vi "Sequence for Constant Dragging with dragging.vi"() -> ()   [LabVIEW 2011]
doc: "The Sequence VI acquires a sequence of images and displays the images in an image control using high-level acquisition VIs. A sequence is appropriate for applications in which you want to process multiple images."
uses:
  <vilib>/userDefined/High Color/IMAQdx.ctl
  <vilib>/vision/driver/IMAQdx.llb/IMAQdx Acquisition Mode.ctl
  <vilib>/Platform/TimedLoop/XDataNode/timing_clust.ctl
  <vilib>/Platform/TimedLoop/XDataNode/nitl_modes.ctl
  <vilib>/Platform/TimedLoop/XDataNode/wakeup.ctl
  <vilib>/vision/driver/IMAQdx.llb/IMAQdx Buffer Number Mode.ctl
  <vilib>/Platform/TimedLoop/XDataNode/XDataNode.xnode
  <vilib>/vision/driver/NI_Vision_Acquisition_Software.lvlib
  Program Files/National Instruments/LabVIEW 2011/resource/objmgr/imaqdx.rc
  <vilib>/Platform/TimedLoop/XDataNode/XDNodeRunTimeDep.lvlib
  Program Files/Mad City Labs/NanoDrive/Madlib.dll
panel:
  in  "Drag Speed (um/s)":dbl min=0.0 step=0.01 format="%_3g"
  in  "Handle 2":i32
  in  "Exposure (us)":dbl(slide)=1407.017543859649 min=100.0 max=15000.0 step=100.0 scale=100.0..15000.0
  out "Acquisition  progress":i32(slide) scale=0.0..10999.0
  in  "BitsPerPixel":u32(ring) items=["Use Hardware Value"=0, "10-bit"=10, "12-bit"=12, "14-bit"=14, "16-bit"=16]
  in  "Height":u32=1080
  in  "Width":u32=1920
  in  "Number of Frames":u32=250
  in  "Frame Rate":dbl=55.0
  in  "Path":path
  in  "Camera Name":T1
  out "Image Array":T2[](array[plugin-control])
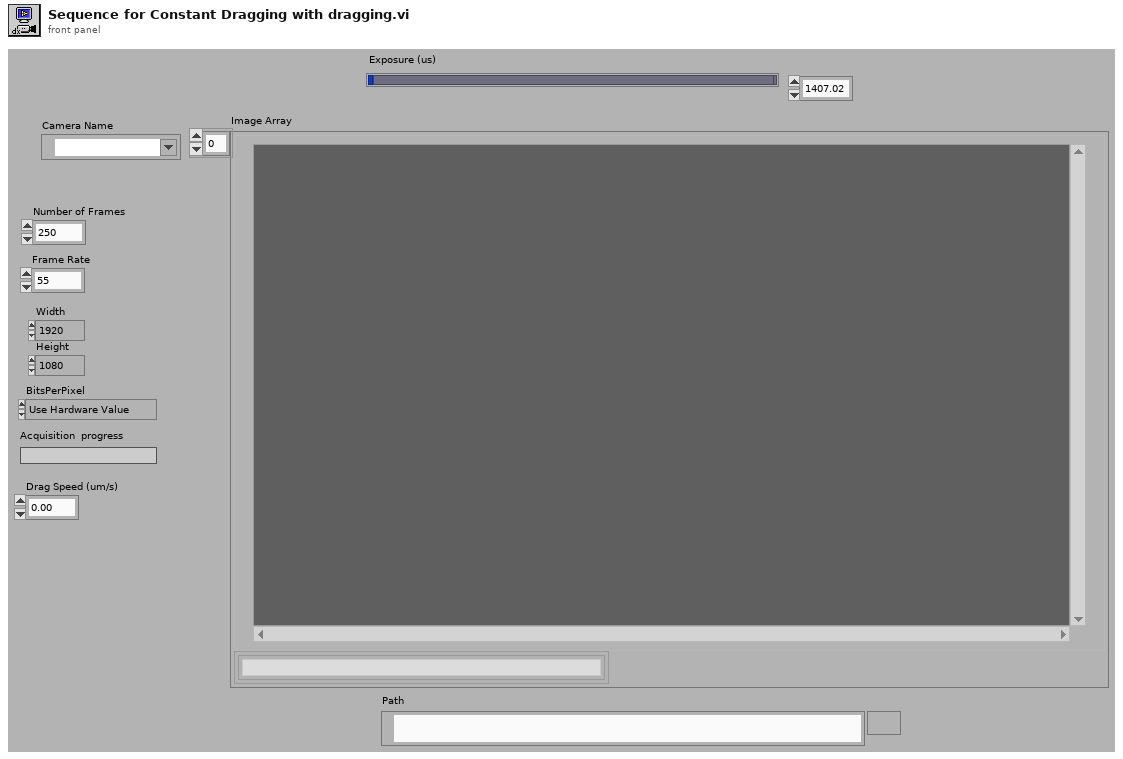
[diagram p1: front panel]
types:
  T1 = typedef "IMAQdx.ctl" = refnum<k21>
  T2 = typedef "IMAQ Image.ctl" = refnum<image>
  T3 = typedef "NI_Vision_Acquisition_Software.lvlib/IMAQdx Acquisition Mode.ctl" = enum32{"One Shot", "Continuous"}
  T4 = typedef "XDNodeRunTimeDep.lvlib/timing_clust.ctl" = cluster{"Expected End [f-1]":u64, "Actual End [f-1]":u64, "Finished Late? [f-1]":bool, "Expected End [i-1]":u64, "Actual End [i-1]":u64, "Finished Late? [i-1]":bool, "Expected Start [i]":u64, "Actual Start [i]":u64, "Expected Start [f]":u64, "Actual Start [f]":u64, "Source Name":string, "Structure Name":string, "Period":i64, "Deadline":i64, "Offset":i64, "Start":i64, "Priority":i32, "Timeout":i32, "Mode":T5, "Wakeup Reason":T6, "Error":errorcluster, "Source Type":string, "Secondary Source Type":string, "Global End Time":u64, "Global Start Time":u64, "Frame Duration":u64, "Iteration Duration":u64, "Assigned CPU":i32, "I/O Scan Engine Mode":u32}
  T5 = typedef "XDNodeRunTimeDep.lvlib/nitl_modes.ctl" = enum32{"No Change", "Process missed periods, maintain original phase", "Discard missed periods, maintain original phase", "Process missed periods, ignore original phase", "Discard missed periods, ignore original phase"}
  T6 = typedef "XDNodeRunTimeDep.lvlib/wakeup.ctl" = enum32{"Normal", "Aborted", "Asynchronous wakeup", "Timing source error", "Timed loop error", "Timeout"}
  T7 = typedef "NI_Vision_Acquisition_Software.lvlib/IMAQdx Buffer Number Mode.ctl" = enum32{"Next", "Last", "Buffer Number"}
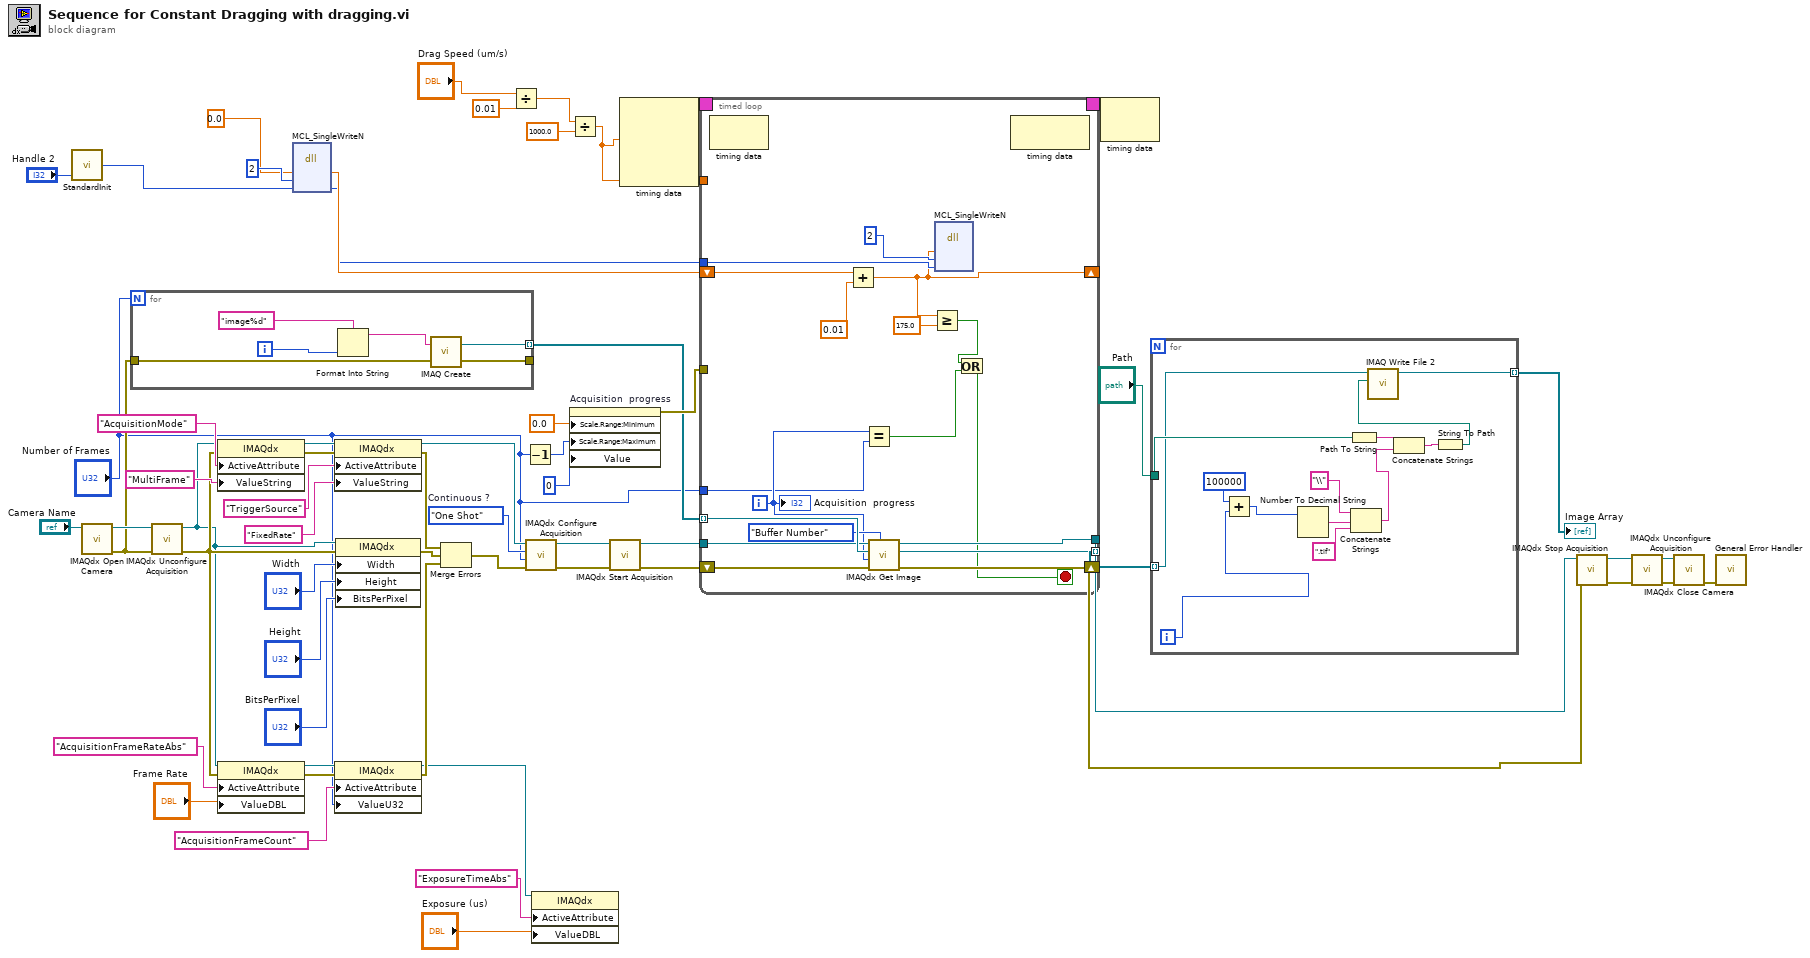
[diagram p0: block diagram]
diagram:
  w38 = IMAQdx_Acquisition_Mode."One Shot"  # Continuous ?
  n1 = call "StandardInit.vi"("Incoming Handle"="Handle 2") -> ("Outgoing Handle"=w11:i32)
  n2 = call <vilib>:"IMAQdx Open Camera.vi"("Session In"="Camera Name") -> ("error out"=w48:errorcluster, "Session Out"=w49:T1)  [unwired: 2 in, 7 out]
  n3 = for {
    N: "Number of Frames" -> [_]
    tunnel: w48 -> [w67]
    tunnel: [w66] -> w26 mode=indexing
    tunnel: [w65] -> _
    i -> [w64]
    n4 = Format Into String(format string="image%d" ("Image Name"), w64) -> (resulting string=w63:string)  [unwired: 2 in, 1 out]
    n5 = call "IMAQ Create"("Image Name"=w63, "error in (no error)"=w67) -> ("New Image"=w66:T2, "error out"=w65:errorcluster)  [unwired: 2 in, 1 out]
  }
  n6 = call <vilib>:"IMAQdx Unconfigure Acquisition.vi"("error in"=w48, "Session In"=w49) -> ("error out"=w43:errorcluster, "Session Out"=w40:T1)  [unwired: 8 out]
  n7 = property class="IMAQdx"(reference=w40, error in=w43, "ActiveAttribute"="AcquisitionMode", "ValueString"="MultiFrame") -> (reference out=w44:T1, error out=w54:errorcluster)
  n8 = property class="IMAQdx"(reference=w40, error in=w43, "ActiveAttribute"="AcquisitionFrameRateAbs", "ValueDBL"="Frame Rate") -> (reference out=w58:T1, error out=w57:errorcluster)
  n9 = dll-call lib="C:/Program Files/Mad City Labs/NanoDrive/Madlib.dll" fn="MCL_SingleWriteN"("position"=0.0, "axis"=u32 2, "handle"=w11) -> ("position"=w5:dbl, "handle"=w4:i32)  [unwired: 4 in, 3 out]
  n10 = property class="IMAQdx"(reference=w44, error in=w54, "ActiveAttribute"="TriggerSource", "ValueString"="FixedRate") -> (reference out=w25:T1, error out=w50:errorcluster)
  n11 = property class="IMAQdx"(reference=w58, error in=w57, "ActiveAttribute"="AcquisitionFrameCount", "ValueU32"="Number of Frames") -> (reference out=w15:T1, error out=w51:errorcluster)
  n12 = property class="IMAQdx"(reference=w40, error in=w43, "Width"="Width", "Height"="Height", "BitsPerPixel"="BitsPerPixel") -> (error out=w42:errorcluster)  [unwired: 1 out]
  n13 = Merge Errors(w50, w42, w51) -> (w22:errorcluster)
  n14 = Divide(x="Drag Speed (um/s)", y=0.01) -> (x/y=w7:dbl)
  n15 = Decrement(x="Number of Frames") -> (x-1=w35:u32)
  n16 = call <vilib>:"IMAQdx Configure Acquisition.vi"("error in"=w22, "Number of Buffers"="Number of Frames", "Continuous?"=w38, "Session In"=w25) -> ("error out"=w21:errorcluster, "Session Out"=w24:T1)  [unwired: 6 out]
  n17 = property class="IMAQdx"(reference=w15, "ActiveAttribute"="ExposureTimeAbs", "ValueDBL"="Exposure (us)") -> ()  [unwired: 1 in, 2 out]
  n18 = Divide(x=w7, y=1000.0) -> (x/y=w1:dbl)
  n19 = property on="Acquisition  progress" class="Slide (strict)"("Scale.Range:Minimum"=0.0 ("Write Attribute"), "Scale.Range:Maximum"=w35, "Value"=u32 0 ("Acquisition  progress")) -> (error out=w27:errorcluster)  [unwired: 2 in, 1 out]
  n20 = call <vilib>:"IMAQdx Start Acquisition.vi"("error in"=w21, "Session In"=w24) -> ("error out"=w37:errorcluster, "Session Out"=w23:T1)  [unwired: 8 out]
  n21 = node-c288(w1) -> (w3:T4)  [unwired: 3 in]
  n22 = timed-loop {
    tunnel: w26 -> [w85] mode=indexing
    shift-right: [w83] -> w34
    shift-left: w37 -> [w84]
    tunnel: [w82] -> w33
    tunnel: w23 -> [w81]
    tunnel: [w79] -> w19 mode=indexing
    tunnel: w27 -> [_]
    tunnel: "Number of Frames" -> [w77]
    tunnel: w1 -> [_]
    tunnel: w4 -> [w76]
    timing: w3 -> [_]
    timing-out: [_] -> w2
    shift-right: [w71] -> _
    shift-left: w5 -> [w75]
    i -> [w78]
    stop <- w68 stop-if-true
    n23 = node-c288() -> ()  [unwired: 1 in, 1 out]
    n24 = Add(x=w75, y=0.01) -> (x+y=w71:dbl)
    n25 = Equal?(x=w78, y=w77) -> (x = y?=w69:bool)
    n26 = call <vilib>:"IMAQdx Get Image.vi"("Buffer Number Mode (Next)"=IMAQdx_Buffer_Number_Mode."Buffer Number", "error in"=w84, "Buffer Number In"=w78, "Image In"=w85, "Session In"=w81) -> ("error out"=w83:errorcluster, "Image Out"=w79:T2, "Session Out"=w82:T1)  [unwired: 4 out]
    n27 = Greater Or Equal?(x=w71, y=175.0) -> (x >= y?=w70:bool)
    n28 = dll-call lib="C:/Program Files/Mad City Labs/NanoDrive/Madlib.dll" fn="MCL_SingleWriteN"("position"=w71, "axis"=u32 2, "handle"=w76) -> ()  [unwired: 6 in, 3 out]
    n29 = Or(x=w70, y=w69) -> (x .or. y?=w68:bool)
    n30 = node-c288() -> ()  [unwired: 1 in, 1 out]
    "Acquisition  progress" <- w78
  }
  n31 = node-c288(w2) -> ()  [unwired: 1 out]
  n32 = for {
    tunnel: "Path" -> [w90]
    tunnel: w19 -> [w89] mode=indexing
    tunnel: [w88] -> w18 mode=indexing
    i -> [w95]
    n33 = Add(x=100000, y=w95) -> (x+y=w97:i32)
    n34 = Number To Decimal String(number=w97) -> (decimal integer string=w100:string)  [unwired: 1 out]
    n35 = Path To String(path=w90) -> (string=w94:string)
    n36 = Concatenate Strings("\\" ("string"), w100, ".tif") -> (w92:string)
    n37 = Concatenate Strings(w94, w92) -> (w93:string)
    n38 = String To Path(string=w93) -> (path=w91:path)
    n39 = call-poly "IMAQ Write File 2"("File Path"=w91, "Image"=w89) -> ("Image Out (duplicate)"=w88:T2)  [unwired: 3 in, 6 out]
  }
  "Image Array" <- w18
  n40 = call <vilib>:"IMAQdx Stop Acquisition.vi"("error in"=w34, "Session In"=w33) -> ("error out"=w32:errorcluster, "Session Out"=w31:T1)  [unwired: 8 out]
  n41 = call <vilib>:"IMAQdx Unconfigure Acquisition.vi"("error in"=w32, "Session In"=w31) -> ("error out"=w30:errorcluster, "Session Out"=w29:T1)  [unwired: 8 out]
  n42 = call <vilib>:"IMAQdx Close Camera.vi"("error in"=w30, "Session In"=w29) -> ("error out"=w39:errorcluster)  [unwired: 9 out]
  n43 = call <vilib>:"General Error Handler.vi"("error in (no error)"=w39) -> ()  [unwired: 1 in, 14 out]
